vi "test_polarplot.vi"() -> ()   [LabVIEW 2019]
panel:
  in  "deg_gps":dbl
  out "2D Picture":picture
  in  "dt":u32=100
  in  "정지":bool
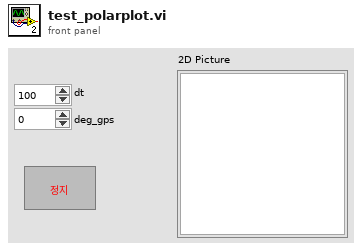
[diagram p1: front panel]
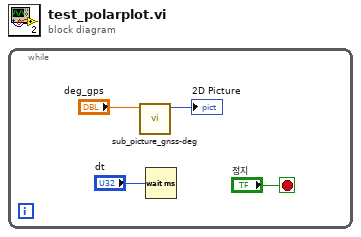
[diagram p0: block diagram]
diagram:
  n1 = while {
    stop <- "정지" stop-if-true
    n2 = call "sub_picture_gnss-deg.vi"("deg_gps"="deg_gps") -> ("new picture"=→"2D Picture":picture)  [unwired: 10 in]
    n3 = Wait (ms)(milliseconds to wait="dt") -> ()  [unwired: 1 out]
  }
